vi "_12_Sample_qsns_03[22].vi"() -> ()   [LabVIEW 2020]
panel:
  out "x*y":i32
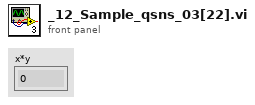
[diagram p1: front panel]
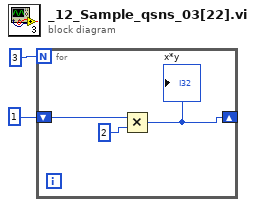
[diagram p0: block diagram]
diagram:
  n1 = for {
    N: 3 -> [_]
    shift-right: [w3] -> _
    shift-left: 1 -> [w5]
    n2 = Multiply(x=w5, y=2) -> (x*y=w3:i32)
    "x*y" <- w3
  }
